vi "2B_Tech_TCP_Packet_CABOZO_v1.vi"(7 "TCP Packet In":string, 12 "Data Array":string[](array[string])) -> (8 "TCP Binary Packet":string)   [LabVIEW 2014]
panel:
  out "array":string[](array[string])
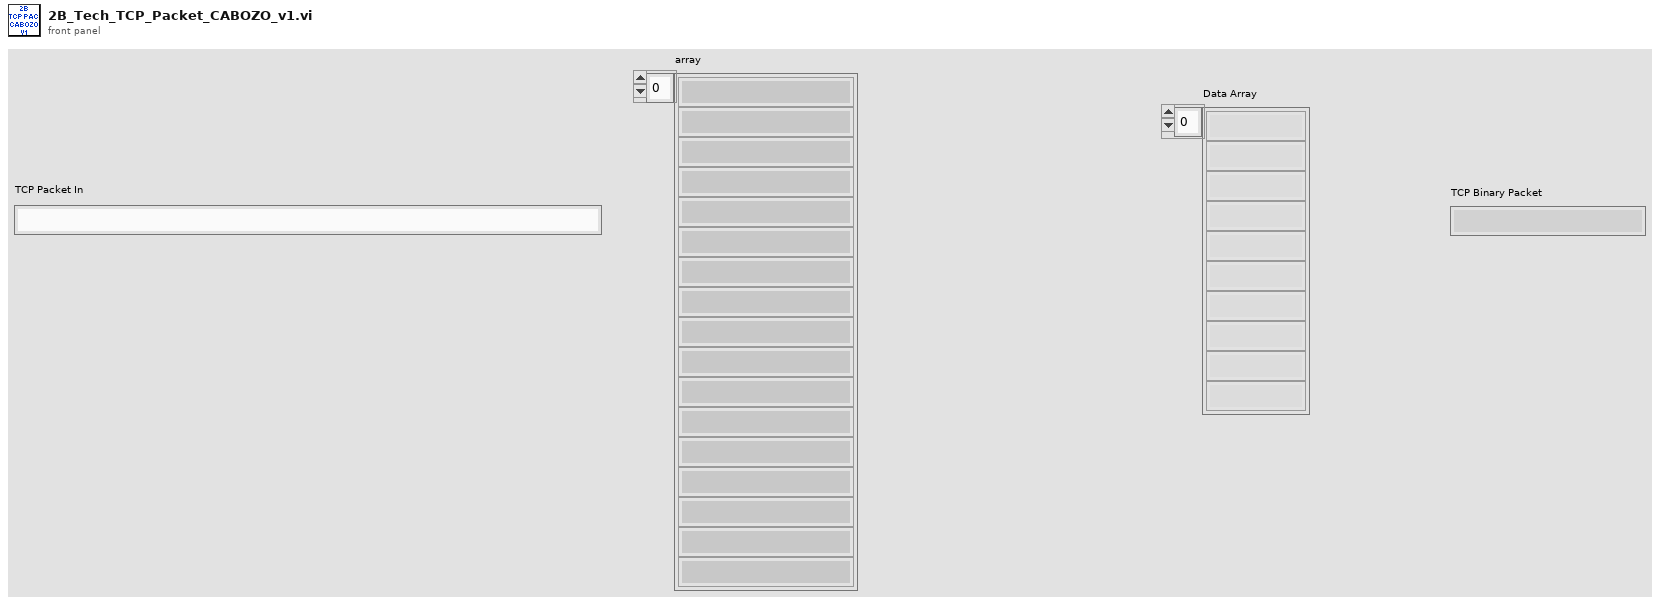
[diagram p1: front panel]
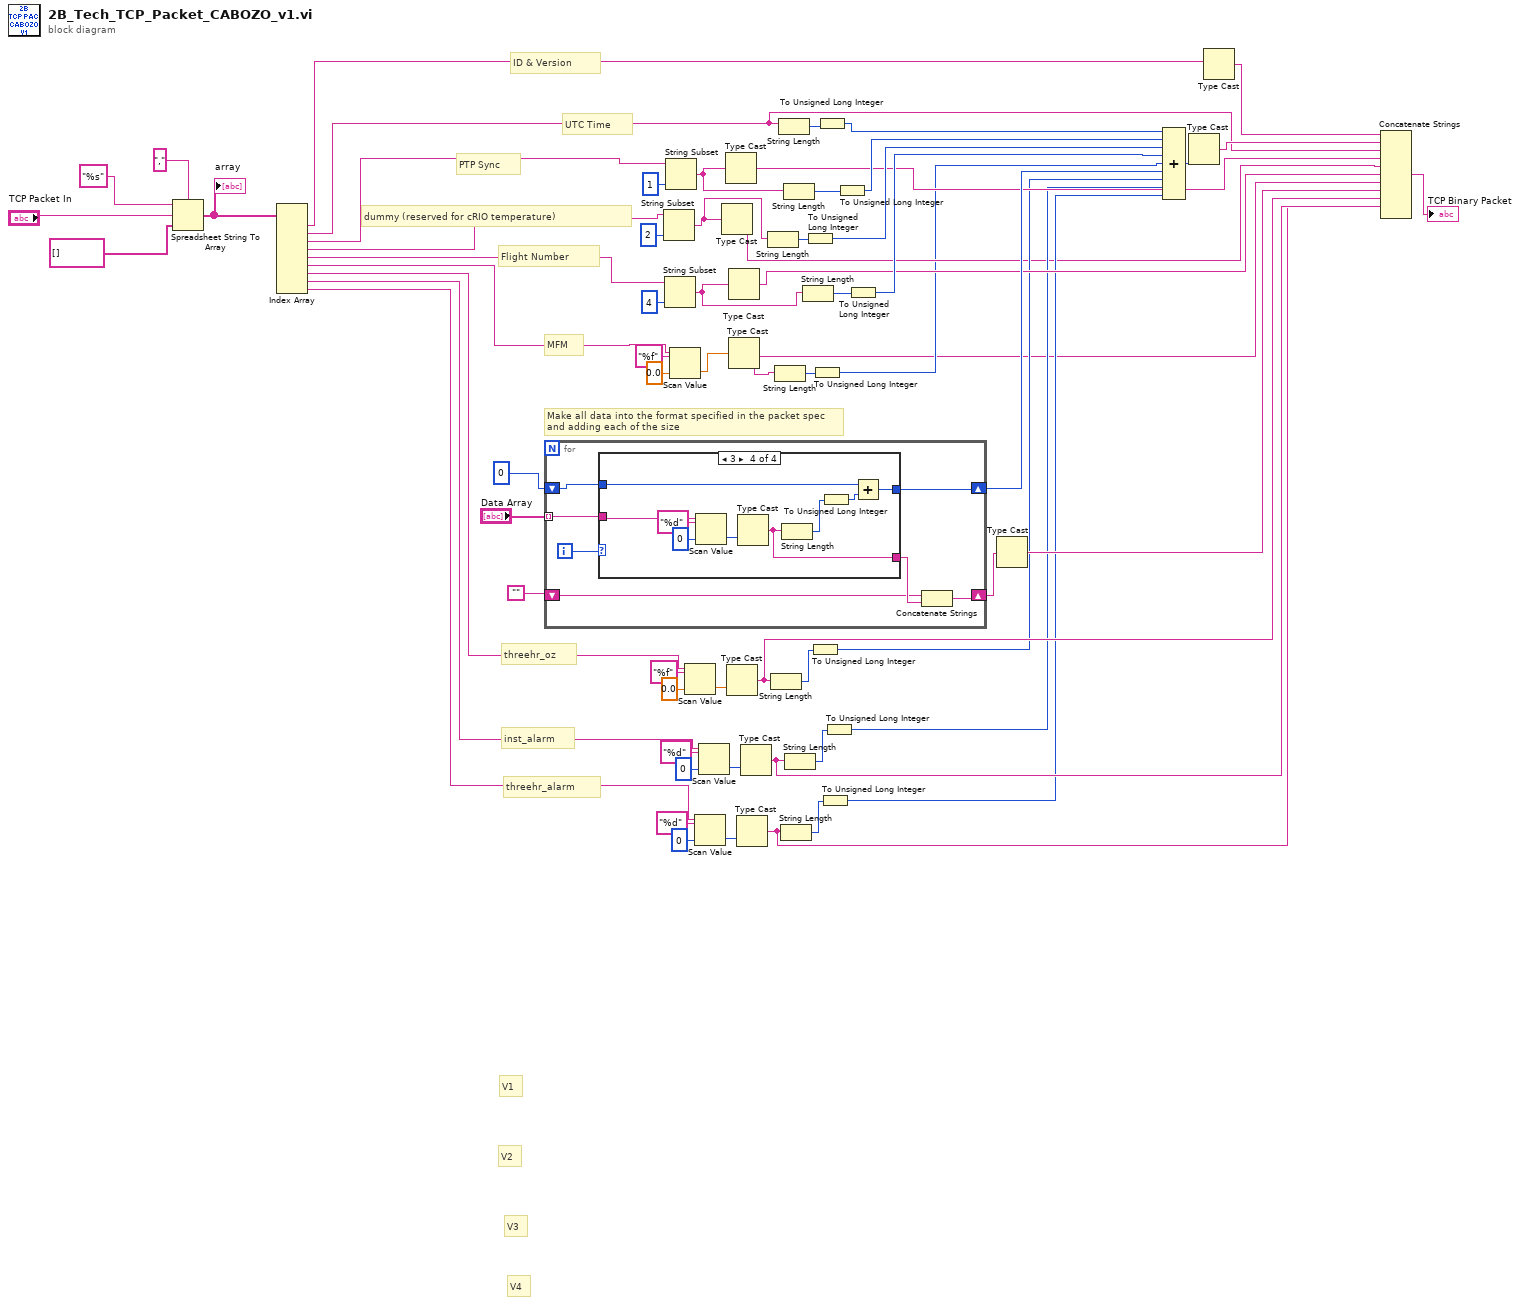
[diagram p0: block diagram]
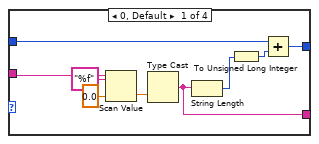
[diagram p2: hidden frame]
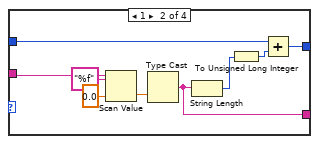
[diagram p3: hidden frame]
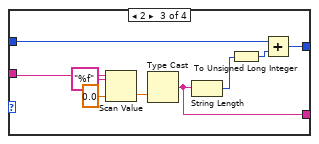
[diagram p4: hidden frame]
diagram:
  # "dummy (reserved for cRIO temperature)"
  # "V4"
  # "V3"
  # "V2"
  # "V1"
  # "threehr_alarm"
  # "inst_alarm"
  # "threehr_oz"
  # "Flight Number"
  # "MFM"
  # "PTP Sync"
  # "UTC Time"
  # "ID & Version"
  # "Make all data into the format specified in the packet spec\nand adding each of the size"
  n1 = Spreadsheet String To Array(delimiter (Tab)=",", format string="%s", spreadsheet string="TCP Packet In", array type (2D Dbl)=string[] []) -> (array=w25:string[])
  "array" <- w25
  n2 = Index Array(array=w25) -> (element #1=w24:string, element #2=w23:string, element #3=w22:string, element #4=w2:string, element #5=w21:string, element #6=w6:string, element #7=w11:string, element #8=w12:string, element #9=w13:string)  [unwired: 9 in]
  n3 = for {
    tunnel: "Data Array" -> [w71] mode=indexing
    shift-right: [w69] -> w53
    shift-left: u32 0 -> [w70]
    shift-right: [w68] -> w42
    shift-left: "" -> [w66]
    i -> [w72]
    n4 = case shown="3" w72 {
      tunnel: w71 -> [w79 w88 w97 w106]
      tunnel: w70 -> [w77 w86 w95 w104]
      tunnel: [w74 w83 w92 w101] -> w69
      tunnel: [w73 w82 w91 w100] -> w67
      frame 0, Default {
        n5 = Scan Value(string=w79, format string="%f", default (0 dbl)=sgl 0.0 ("default (0 I32)")) -> (value=w81:sgl)  [unwired: 1 out]
        n6 = Type Cast(x=w81) -> (*(type *) &x=w73:string)  [unwired: 1 in]
        n7 = String Length(string=w73) -> (length=w76:i32)
        n8 = To Unsigned Long Integer(number=w76) -> (unsigned 32bit integer=w75:u32)
        n9 = Add(x=w77, y=w75) -> (x+y=w74:u32)
      }
      frame 1 {
        n10 = Scan Value(string=w88, format string="%f", default (0 dbl)=sgl 0.0 ("default (0 I32)")) -> (value=w90:sgl)  [unwired: 1 out]
        n11 = Type Cast(x=w90) -> (*(type *) &x=w82:string)  [unwired: 1 in]
        n12 = String Length(string=w82) -> (length=w85:i32)
        n13 = To Unsigned Long Integer(number=w85) -> (unsigned 32bit integer=w84:u32)
        n14 = Add(x=w86, y=w84) -> (x+y=w83:u32)
      }
      frame 2 {
        n15 = Scan Value(string=w97, format string="%f", default (0 dbl)=sgl 0.0 ("default (0 I32)")) -> (value=w99:sgl)  [unwired: 1 out]
        n16 = Type Cast(x=w99) -> (*(type *) &x=w91:string)  [unwired: 1 in]
        n17 = String Length(string=w91) -> (length=w94:i32)
        n18 = To Unsigned Long Integer(number=w94) -> (unsigned 32bit integer=w93:u32)
        n19 = Add(x=w95, y=w93) -> (x+y=w92:u32)
      }
      frame 3 {
        n20 = Scan Value(string=w106, format string="%d", default (0 dbl)=0 ("default (0 I32)")) -> (value=w108:i32)  [unwired: 1 out]
        n21 = Type Cast(x=w108) -> (*(type *) &x=w100:string)  [unwired: 1 in]
        n22 = String Length(string=w100) -> (length=w103:i32)
        n23 = To Unsigned Long Integer(number=w103) -> (unsigned 32bit integer=w102:u32)
        n24 = Add(x=w104, y=w102) -> (x+y=w101:u32)
      }
    }
    n25 = Concatenate Strings(w66, w67) -> (w68:string)
  }
  n26 = String Subset(string=w2, length (rest)=2 ("length (rest)")) -> (substring=w1:string)  [unwired: 1 in]
  n27 = String Subset(string=w21, length (rest)=4 ("length (rest)")) -> (substring=w46:string)  [unwired: 1 in]
  n28 = String Subset(string=w22, length (rest)=1 ("length (rest)")) -> (substring=w49:string)  [unwired: 1 in]
  n29 = Scan Value(string=w6, format string="%f", default (0 dbl)=sgl 0.0 ("default (0 I32)")) -> (value=w7:sgl)  [unwired: 1 out]
  n30 = Scan Value(string=w11, format string="%f", default (0 dbl)=sgl 0.0 ("default (0 I32)")) -> (value=w41:sgl)  [unwired: 1 out]
  n31 = Scan Value(string=w13, format string="%d", default (0 dbl)=u16 0 ("default (0 I32)")) -> (value=w20:u16)  [unwired: 1 out]
  n32 = Scan Value(string=w12, format string="%d", default (0 dbl)=u16 0 ("default (0 I32)")) -> (value=w35:u16)  [unwired: 1 out]
  n33 = Type Cast(x=w1) -> (*(type *) &x=w14:string)  [unwired: 1 in]
  n34 = Type Cast(x=w49) -> (*(type *) &x=w48:string)  [unwired: 1 in]
  n35 = Type Cast(x=w41) -> (*(type *) &x=w37:string)  [unwired: 1 in]
  n36 = Type Cast(x=w46) -> (*(type *) &x=w47:string)  [unwired: 1 in]
  n37 = Type Cast(x=w7) -> (*(type *) &x=w4:string)  [unwired: 1 in]
  n38 = Type Cast(x=w20) -> (*(type *) &x=w15:string)  [unwired: 1 in]
  n39 = Type Cast(x=w35) -> (*(type *) &x=w30:string)  [unwired: 1 in]
  n40 = String Length(string=w1) -> (length=w60:i32)
  n41 = String Length(string=w37) -> (length=w38:i32)
  n42 = String Length(string=w4) -> (length=w10:i32)
  n43 = String Length(string=w23) -> (length=w65:i32)
  n44 = String Length(string=w15) -> (length=w17:i32)
  n45 = String Length(string=w49) -> (length=w62:i32)
  n46 = String Length(string=w30) -> (length=w32:i32)
  n47 = String Length(string=w46) -> (length=w57:i32)
  n48 = To Unsigned Long Integer(number=w60) -> (unsigned 32bit integer=w59:u32)
  n49 = To Unsigned Long Integer(number=w38) -> (unsigned 32bit integer=w36:u32)
  n50 = To Unsigned Long Integer(number=w10) -> (unsigned 32bit integer=w5:u32)
  n51 = To Unsigned Long Integer(number=w65) -> (unsigned 32bit integer=w64:u32)
  n52 = To Unsigned Long Integer(number=w17) -> (unsigned 32bit integer=w16:u32)
  n53 = To Unsigned Long Integer(number=w32) -> (unsigned 32bit integer=w31:u32)
  n54 = To Unsigned Long Integer(number=w62) -> (unsigned 32bit integer=w61:u32)
  n55 = To Unsigned Long Integer(number=w57) -> (unsigned 32bit integer=w56:u32)
  n56 = Type Cast(x=w42) -> (*(type *) &x=w45:string)  [unwired: 1 in]
  n57 = Compound Arithmetic op=ADD(w64, w61, w59, w56, w5, w53, w36, w31, w16) -> (w51:u32)
  n58 = Type Cast(x=w51) -> (*(type *) &x=w50:string)  [unwired: 1 in]
  n59 = Type Cast(x=w24) -> (*(type *) &x=w52:string)  [unwired: 1 in]
  n60 = Concatenate Strings(w52, w50, w23, w48, w14, w47, w4, w45, w37, w30, w15) -> (→"TCP Binary Packet":string)
